vi "LineStyle.vi"(1 "Enum LineStyle":u16) -> (0 "LineStyle":string)   [LabVIEW 2025]
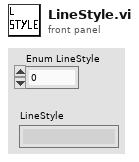
[diagram p1: front panel]
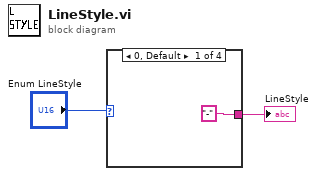
[diagram p0: block diagram]
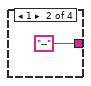
[diagram p2: hidden frame]
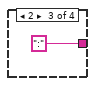
[diagram p3: hidden frame]
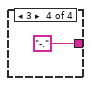
[diagram p4: hidden frame]
diagram:
  n1 = case shown="0, Default" "Enum LineStyle" {
    tunnel: ["-" "--" ":" "-."] -> w2
    frame 0, Default {
    }
    frame 1 {
    }
    frame 2 {
    }
    frame 3 {
    }
  }
  "LineStyle" <- w2
